vi "Run.vi"(8 "error in (no error)":errorcluster, 11 "Timer Demo App in":refnum<class "Timer Demo App.lvclass">) -> (0 "error out":errorcluster, 3 "Timer Demo App out":refnum<class "Timer Demo App.lvclass">)   [LabVIEW 2020, in "Timer Demo.lvlib" / "Timer Demo App.lvclass"]
uses:
  Timer Demo App.lvclass
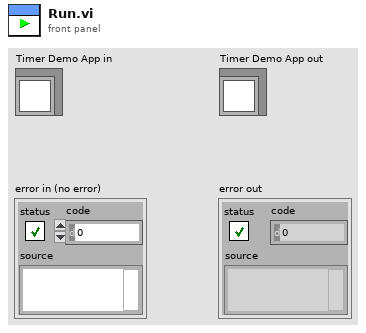
[diagram p1: front panel]
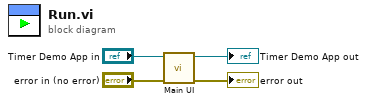
[diagram p0: block diagram]
diagram:
  n1 = call "Main UI.vi"("error in (no error)"="error in (no error)", "Timer Demo App in"="Timer Demo App in") -> ("error out"=→"error out":errorcluster, "Timer Demo App out"=→"Timer Demo App out":refnum<class "Timer Demo App.lvclass">)  [unwired: 8 in]
